vi "V1_moveby_inputs.vi"(4 "mounts":T1={"mount labels"=["Mount 1", "Mount 2", "Mount 3", "Mount 4"], "mount inputs"=[]}, 5 "channel pairs":cluster{i32, i32}[](array[cluster]), 11 "Voltage Array in":refnum<vi>) -> (6 "case selector":i16[](array[numeric]), 9 "even channels":i32[](array[numeric]), 10 "odd channels":i32[](array[numeric]))   [LabVIEW 2020]
panel:
  out "channel pairs 2":cluster{i32, i32}[](array[cluster])
  out "0, 2":i16[](array[numeric])
  out "0, 1":i16[](array[numeric])
  out "In Range? 2":bool[](array[boolean])
  out "In Range?":bool[](array[boolean])
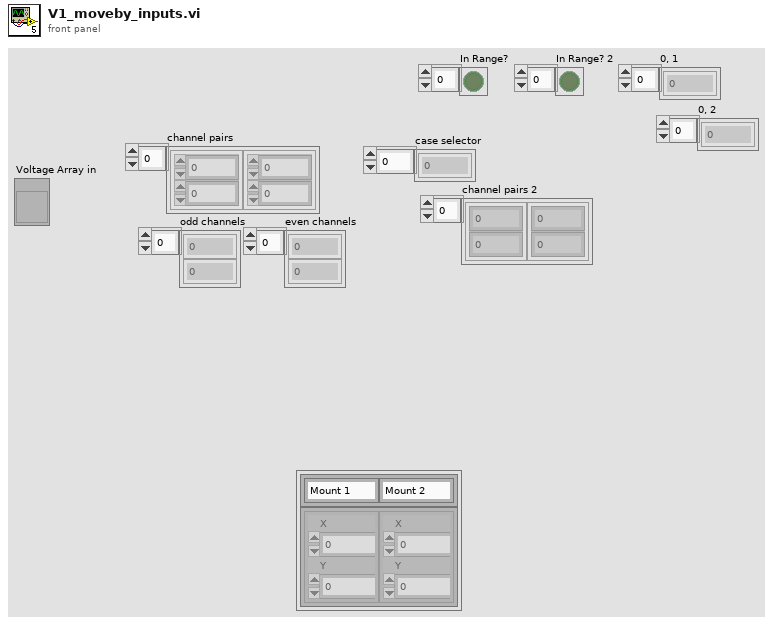
[diagram p1: front panel]
types:
  T1 = cluster{"mount labels":string[], "mount inputs":cluster{"X":dbl, "Y":dbl}[]}
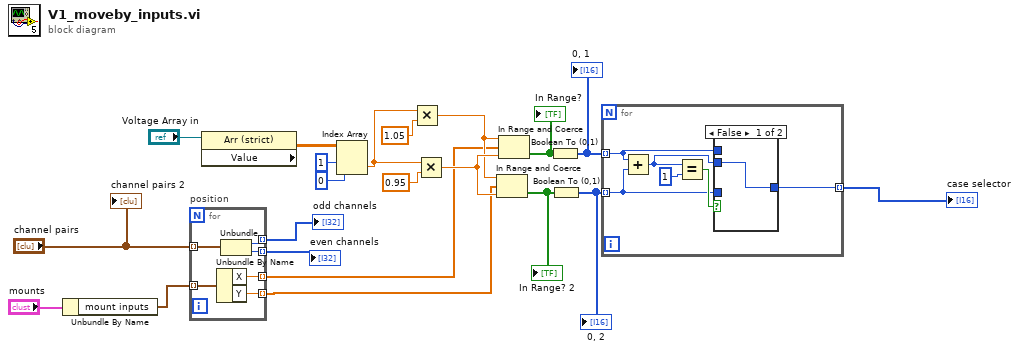
[diagram p0: block diagram]
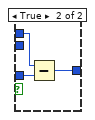
[diagram p2: hidden frame]
diagram:
  n1 = Unbundle By Name("mounts") -> ("mount inputs"=w8:cluster{"X":dbl, "Y":dbl}[])
  n2 = for "position" {
    tunnel: w8 -> [w27] mode=indexing
    tunnel: [w26] -> w15 mode=indexing
    tunnel: [w25] -> w19 mode=indexing
    tunnel: "channel pairs" -> [w24] mode=indexing
    tunnel: [w23] -> w5 mode=indexing
    tunnel: [w22] -> w4 mode=indexing
    n3 = Unbundle By Name(w27) -> ("X"=w26:dbl, "Y"=w25:dbl)
    n4 = Unbundle(w24) -> (w23:i32, w22:i32)
  }
  "odd channels" <- w5
  "even channels" <- w4
  n5 = property class="Arr (strict)"(reference="Voltage Array in") -> ("Value"=w10:dbl[][])  [unwired: 1 in, 2 out]
  n6 = Index Array(array=w10, index (row)=1, index (col)=0 ("disabled index (col)")) -> (element=w18:dbl)
  n7 = Multiply(x=w18, y=1.05) -> (x*y=w20:dbl)
  n8 = Multiply(x=w18, y=0.95) -> (x*y=w21:dbl)
  n9 = In Range and Coerce(upper limit=w20, x=w19, lower limit=w21) -> (In Range?=w13:bool[])  [unwired: 1 out]
  "In Range? 2" <- w13
  n10 = In Range and Coerce(upper limit=w20, x=w15, lower limit=w21) -> (In Range?=w14:bool[])  [unwired: 1 out]
  "In Range?" <- w14
  n11 = Boolean To (0,1)(Boolean=w14) -> (0, 1=w11:i16[])
  "0, 1" <- w11
  n12 = Boolean To (0,1)(Boolean=w13) -> (0, 1=w12:i16[])
  "0, 2" <- w12
  n13 = for {
    tunnel: w11 -> [w29] mode=indexing
    tunnel: w12 -> [w30] mode=indexing
    tunnel: [w28] -> w1 mode=indexing
    n14 = Add(x=w29, y=w30) -> (x+y=w31:i16)
    n15 = Equal?(x=w31, y=i16 1) -> (x = y?=w32:bool)
    n16 = case shown="False" w32 {
      tunnel: [w34 w35] -> w28
      tunnel: w31 -> [w34 _]
      tunnel: w30 -> [_ w37]
      tunnel: w29 -> [_ w36]
      frame False {
      }
      frame True {
        n17 = Subtract(x=w36, y=w37) -> (x-y=w35:i16)
      }
    }
  }
  "case selector" <- w1
  "channel pairs 2" <- "channel pairs"
